vi "Get.vi"(8 "error in (no error)":errorcluster, 10 "Key":string, 11 "Dictionary in":refnum<class "Dictionary.lvclass">) -> (0 "error out":errorcluster, 1 "Success?":bool, 2 "Value":variant, 3 "Dictionary out":refnum<class "Dictionary.lvclass">)   [LabVIEW 2018, in "Application.lvlib" / "Dictionary.lvclass"]
uses:
  Dictionary.lvclass
  Dictionary.lvclass/Dictionary.ctl
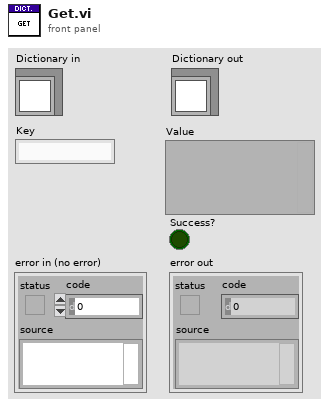
[diagram p1: front panel]
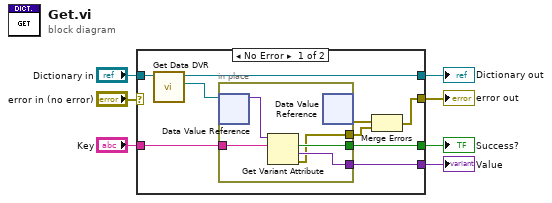
[diagram p0: block diagram]
diagram:
  n1 = case shown="No Error" "error in (no error)" {
    selector: "error in (no error)" -> [_ w23]
    tunnel: [w8 w23] -> w6
    tunnel: [w14 w22] -> w4
    tunnel: "Dictionary in" -> [w16 w22]
    tunnel: "Key" -> [w13 _]
    tunnel: [w12 _] -> w2
    tunnel: [w11 _] -> w1
    frame No Error {
      n2 = call "Get Data DVR.vi"("Dictionary in"=w16) -> ("Data DVR"=w15:refnum<data-value>, "Dictionary out"=w14:refnum<class "Dictionary.lvclass">)  [unwired: 8 in, 1 out]
      n3 = in-place {
        in-place-border: w13 -> [w20]
        in-place-border: [w19] -> w12
        in-place-border: [w18] -> w11
        in-place-border: [w17] -> w9
        n4 = in-place-dvr #1(w15) -> (w21:variant)  [unwired: 1 out]
        n5 = Get Variant Attribute(Variant=w21, name=w20) -> (found=w19:bool, value=w18:variant, error out=w17:errorcluster)  [unwired: 2 in, 1 out]
        n6 = in-place-dvr #1() -> (w10:errorcluster)  [unwired: 1 in, 1 out]
      }
      n7 = Merge Errors(w10, w9) -> (w8:errorcluster)
    }
    frame Error {
    }
  }
  "error out" <- w6
  "Dictionary out" <- w4
  "Success?" <- w2
  "Value" <- w1
